vi "Get SeperatedLayers.vi"(8 "error in (no error)":errorcluster, 11 "DLP2 in":refnum<class "DLP2.lvclass">) -> (0 "error out":errorcluster, 1 "Sorted Heads[]":u8[](array[numeric]), 2 "Images":T1[](array[typedef]), 3 "DLP2 out":refnum<class "DLP2.lvclass">)   [LabVIEW 2022 SP3, in "DLP2.lvclass"]
doc: "Developed by Kevin Thompson\nkevin@thompsonengineering.net\n\nCopyright 2018\nThompson Engineering, LLC"
uses:
  DLP2.lvclass
  <vilib>/vision/Image Controls.llb/IMAQ Image.ctl
  DLP2.lvclass/DLP2.ctl
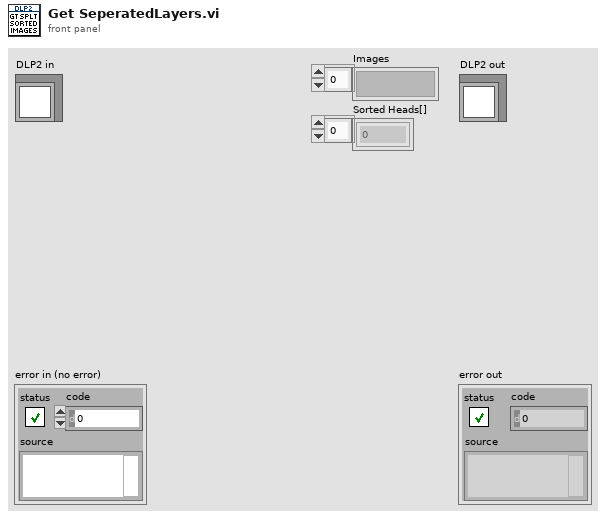
[diagram p1: front panel]
types:
  T1 = typedef "IMAQ Image.ctl" = refnum<image>
  T2 = typedef "DLP2.lvclass/ObjData--cluster.ctl" = cluster{"Settings":T3, "Public Events":T4, "Dependency":T5, "ReadData-placeholder":T6, "VISA-placeholder":refnum<visa-resource-name>, "Images":T1[], "Sorted Heads[]":u8[]}
  T3 = typedef "DLP2.lvclass/Settings--cluster.ctl" = cluster{"Simulation":bool}
  T4 = typedef "DLP2.lvclass/Public Events--cluster.ctl" = cluster{"Temp01.AsyncCmd Event":refnum<user-event>, "Temp01.AsyncMsg Event":refnum<user-event>, "stop process":refnum<user-event>, "API Incoming Event":refnum<user-event>, "API Executed Event":refnum<user-event>, "API Return Event":refnum<user-event>, "Images":refnum<user-event>}
  T5 = typedef "DLP2.lvclass/Dependency--cluster.ctl" = cluster{"Config":refnum<class>, "Database":refnum<class "Database.lvclass">}
  T6 = typedef "DLP2.lvclass/Read Data--cluster.ctl" = cluster{"Data":dbl}
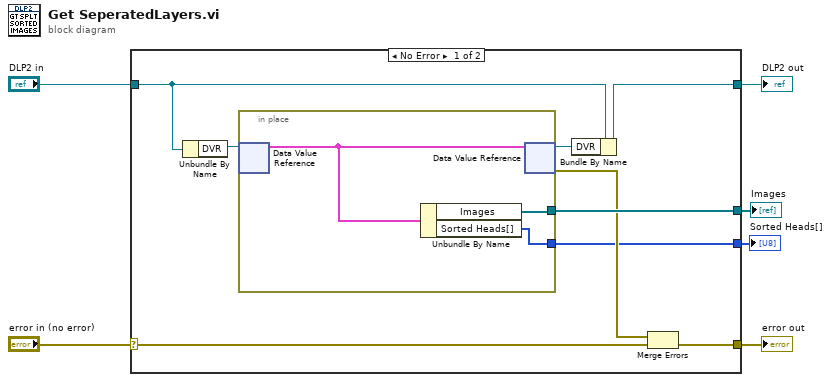
[diagram p0: block diagram]
diagram:
  n1 = case shown="No Error" "error in (no error)" {
    selector: "error in (no error)" -> [w15 w19]
    tunnel: [w9 w19] -> w5
    tunnel: [w11 w20] -> w3
    tunnel: "DLP2 in" -> [w12 w20]
    tunnel: [w10 _] -> w2
    tunnel: [w7 _] -> w1
    frame No Error {
      n2 = Unbundle By Name(w12) -> ("DVR"=w13:refnum<data-value>)
      n3 = in-place {
        in-place-border: [w17] -> w10
        in-place-border: [w16] -> w7
        n4 = in-place-dvr #1(w13) -> (w18:T2)  [unwired: 1 out]
        n5 = Unbundle By Name(w18) -> ("Images"=w17:T1[], "Sorted Heads[]"=w16:u8[])
        n6 = in-place-dvr #1(w18) -> (w14:refnum<data-value>, w8:errorcluster)
      }
      n7 = Bundle By Name(cluster=w12, "DVR"=w14) -> (w11:refnum<class "DLP2.lvclass">)
      n8 = Merge Errors(w8, w15) -> (w9:errorcluster)
    }
    frame Error {
    }
  }
  "error out" <- w5
  "DLP2 out" <- w3
  "Images" <- w2
  "Sorted Heads[]" <- w1
